vi "Init Async Elements.vi"(10 "Async Elements":refnum<queue>) -> (3 "Base Async Elements out":refnum<class "Base Async Elements.lvclass">)   [LabVIEW 2020, in "jettl.lvlib" / "Base Async Elements.lvlib" / "Base Async Elements.lvclass"]
uses:
  Base Async Elements.lvclass
  Base Async Elements.lvclass/Base Async Elements.ctl
  Async Elements.ctl
  jettl.lvlib
  Transport/Transport.lvclass
  Msg/Msg.lvclass
  Msgs.ctl
  Actor/Actor.lvclass
  Attributes Metadata/Attributes Metadata.lvclass
  Attributes.ctl
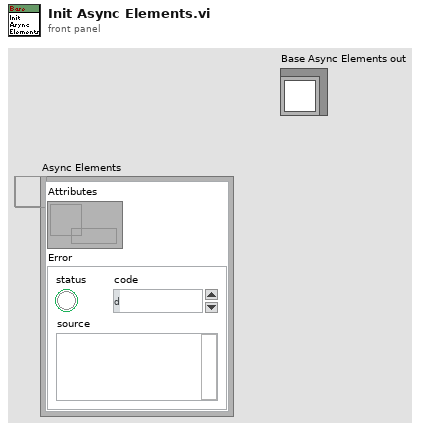
[diagram p1: front panel]
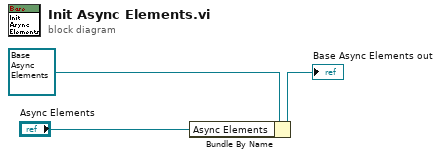
[diagram p0: block diagram]
diagram:
  n1 = Bundle By Name(cluster=refnum<class "Base Async Elements.lvclass"> refnum ("Base Async Elements out"), "Async Elements"="Async Elements") -> (→"Base Async Elements out":refnum<class "Base Async Elements.lvclass">)
